vi "CountAtoms.vi"(0 "Cursor List":T2, 5 "Atom Image":dbl[][](graph), 7 "Experimental Variables":T1={"Pixel Size before binning (µm)"=6.0, "Imaging Wavelength (m)"=4.61e-07, "Isotope"=84, "1P1 Linewidth (MHz)"=30.5, "Imaging Detuning (MHz)"=0.0, "Software Bin Size"=1} {"Software Bin Size" items=["1"=1, "2"=2, "3"=3, "4"=4, "5"=5, "6"=6, "7"=7, "8"=8]; "Isotope" min=84 max=88; "Imaging Wavelength (m)" format="%#_6p"}, 9 "Background Image":dbl[][](graph), 11 "Drop Time":dbl=1e-06 min=1e-06 format="%#_6p") -> (4 "Number":dbl, 6 "OD":dbl[][](graph), 8 "Data Cuts":dbl[][](graph), 10 "Temperature (K) x":dbl format="%#_6p", 15 "Temperature (K) y":dbl format="%#_6p")   [LabVIEW 2015]
uses:
  <vilib>/Utility/miscctls.llb/LVCursorListTypeDef.ctl
  Controls/ExperimentParameters/experimentalvariables.ctl
  <vilib>/Utility/file.llb/Write Delimited Spreadsheet (DBL).vi
  <vilib>/Utility/file.llb/Read Delimited Spreadsheet (DBL).vi
panel:
  out "standard output":string
  out "standard error":string
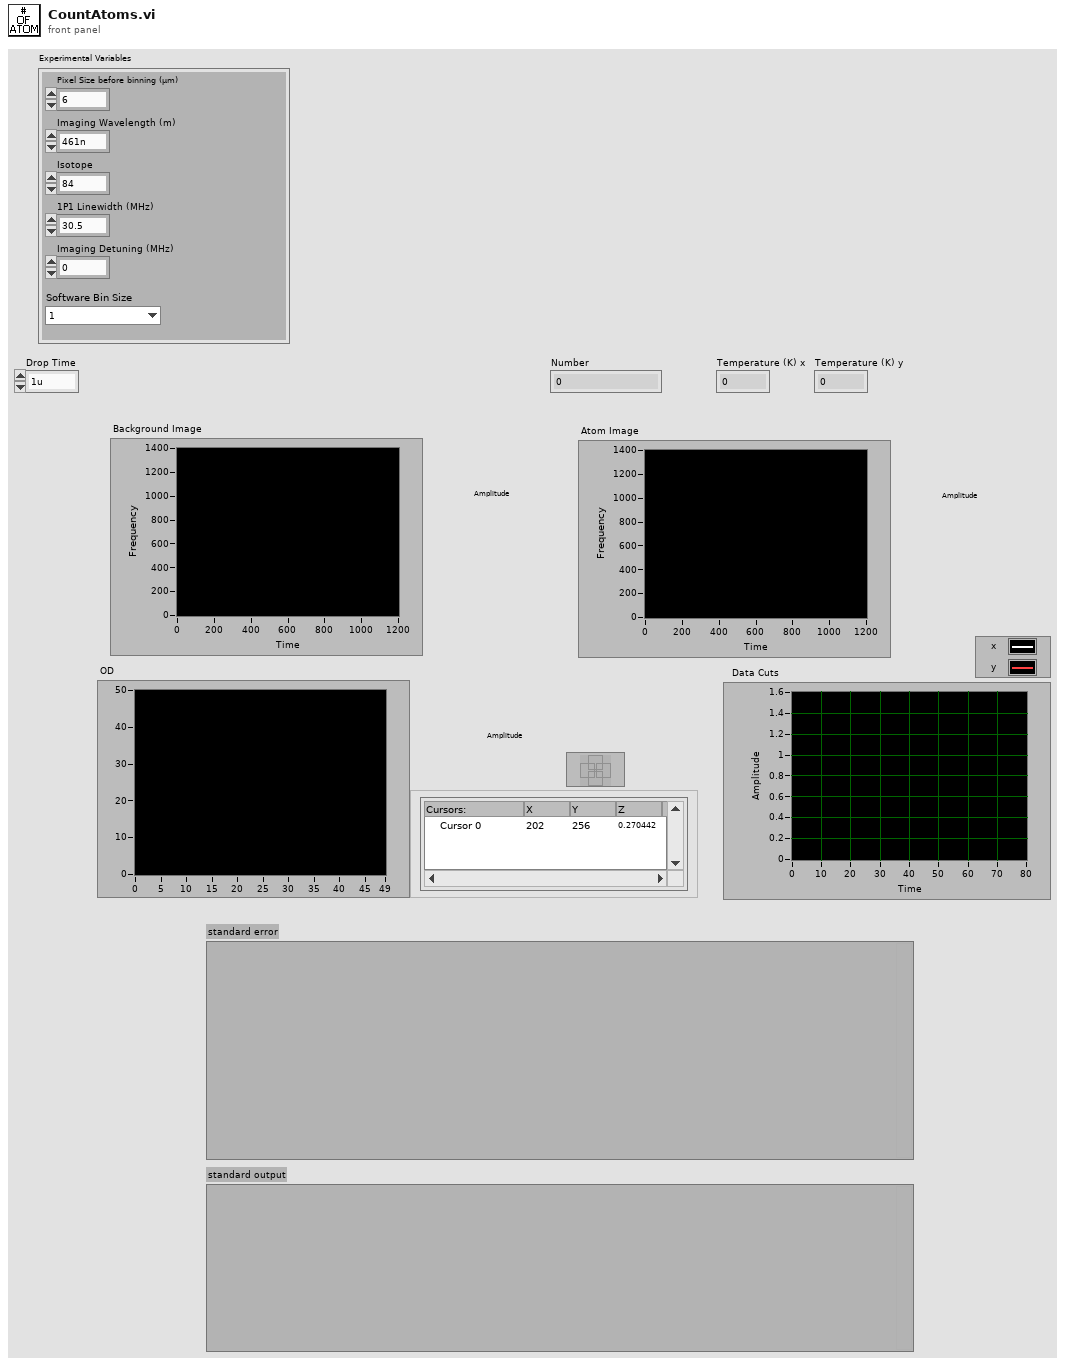
[diagram p1: front panel]
types:
  T1 = typedef "experimentalvariables.ctl" = cluster{"Pixel Size before binning (µm)":dbl, "Imaging Wavelength (m)":dbl, "Isotope":i32, "1P1 Linewidth (MHz)":dbl, "Imaging Detuning (MHz)":dbl, "Software Bin Size":u16}
  T2 = typedef "LVCursorListTypeDef.ctl" = cluster{"Name":string, "Color":u32, "Style":u8, "Point Style":u8, "Name Visible":bool, "Allow Drag":bool, "Cursor Mode":u32, "Plot":i32, "Index":i32, "Position":cluster{"X":dbl, "Y":dbl}, "X Scale":u32, "Y Scale":u32, "Watch Plots":i32[], "Watch All Plots":bool, "Plot Area":i32, "Label Offset":cluster{"X":dbl, "Y":dbl}}[]
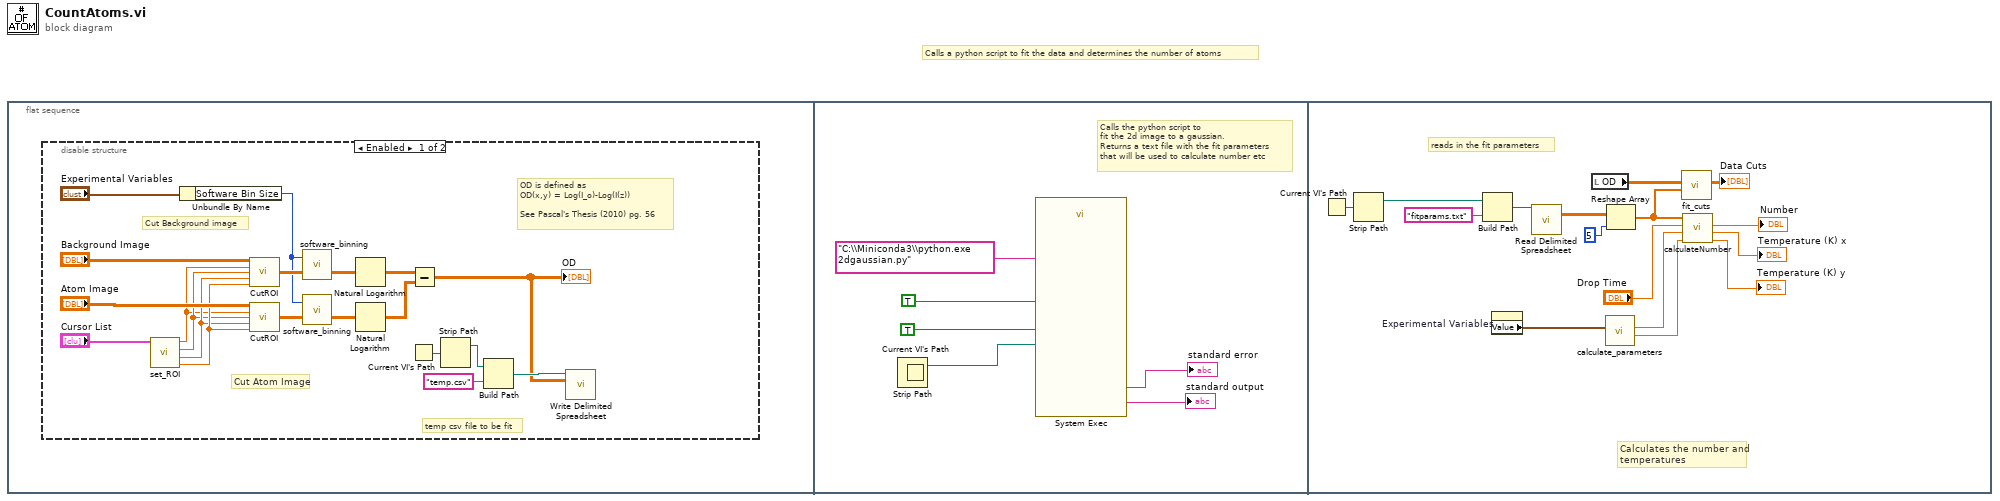
[diagram p0: block diagram]
diagram:
  # "Calls a python script to fit the data and determines the number of atoms"
  n1 = flat-sequence {
    frame #0 {
      n2 = disable-structure shown="Enabled" {
        frame Enabled {
          # "temp csv file to be fit"
          # "OD is defined as \nOD(x,y) = Log(I_o)-Log(I(z))\n\nSee Pascal's Thesis (2010) pg. 56"
          # "Cut Atom Image"
          # "Cut Background image"
          n3 = call "set_ROI.vi"("Cursor List"="Cursor List") -> ("Row End"=w15:dbl, "RowStart"=w14:dbl, "ColEnd"=w13:dbl, "ColStart"=w12:dbl)  [unwired: 7 in]
          n4 = Unbundle By Name("Experimental Variables") -> ("Software Bin Size"=w1:u16)
          n5 = call "CutROI.vi"("Full Image In"="Background Image", "Col Start"=w12, "Col End"=w13, "Row Start"=w14, "Row End"=w15) -> ("Cut Image Out"=w5:dbl[][])  [unwired: 10 in]
          n6 = call "CutROI.vi"("Full Image In"="Atom Image", "Col Start"=w12, "Col End"=w13, "Row Start"=w14, "Row End"=w15) -> ("Cut Image Out"=w3:dbl[][])  [unwired: 10 in]
          n7 = call "software_binning.vi"("Input Array"=w5, "bin size"=w1) -> ("Binned Array"=w4:dbl[][])  [unwired: 1 in]
          n8 = call "software_binning.vi"("Input Array"=w3, "bin size"=w1) -> ("Binned Array"=w2:dbl[][])  [unwired: 1 in]
          n9 = Natural Logarithm(1:w4) -> (0:w17:dbl[][])
          n10 = Natural Logarithm(1:w2) -> (0:w16:dbl[][])
          n11 = Current VI's Path() -> (path=w10:path)
          n12 = Subtract(x=w17, y=w16) -> (x-y=w6:dbl[][])
          "OD" <- w6
          n13 = Strip Path(path=w10) -> (stripped path=w9:path)  [unwired: 1 out]
          n14 = Build Path(base path=w9, name or relative path="temp.csv") -> (appended path=w8:path)
          n15 = call-poly <vilib>:"Write Delimited Spreadsheet.vi"("file path (dialog if empty)"=w8, "2D data"=w6) -> ()  [unwired: 12 in, 2 out]
        }
        frame Disabled {
        }
      }
    }
    frame #1 {
      # "Calls the python script to\nfit the 2d image to a gaussian.\nReturns a text file with the fit parameters\nthat will be used to calculate number etc"
      n16 = Current VI's Path() -> (path=w23:path)
      n17 = Strip Path(path=w23) -> (stripped path=w22:path)  [unwired: 1 out]
      n18 = call <vilib>:"System Exec.vi"("run minimized? (F)"=TRUE, "wait until completion? (T)"=TRUE, "working directory"=w22, "command line"="C:\\Miniconda3\\python.exe 2dgaussian.py") -> ("standard error"=→"standard error":string, "standard output"=→"standard output":string)  [unwired: 4 in, 2 out]
    }
    frame #2 {
      # "Calculates the number and \ntemperatures"
      # "reads in the fit parameters"
      n19 = Current VI's Path() -> (path=w34:path)
      n20 = Strip Path(path=w34) -> (stripped path=w33:path)  [unwired: 1 out]
      n21 = Build Path(base path=w33, name or relative path="fitparams.txt") -> (appended path=w35:path)
      n22 = property on="Experimental Variables" class="Clust (strict)"() -> ("Value"=w30:T1)  [unwired: 2 in, 2 out]
      n23 = call-poly <vilib>:"Read Delimited Spreadsheet.vi"("file path (dialog if empty)"=w35) -> ("all rows"=w43:dbl[][])  [unwired: 9 in, 5 out]
      n24 = local read "OD"() -> (w38:dbl[][])
      n25 = call "calculate_parameters.vi"("Experimental Variables"=w30) -> ("Effective Pixel Size (µm)"=w28:dbl, "Cross Section (m^2)"=w29:dbl)  [unwired: 8 in, 1 out]
      n26 = Reshape Array(w43, 5 ("dimension size")) -> (w31:dbl[])
      n27 = call "fit_cuts.vi"("Array"=w31, "Intensity Graph"=w38) -> ("Waveform Graph"=→"Data Cuts":dbl[][])  [unwired: 9 in]
      n28 = call "calculateNumber.vi"("Array"=w31, "Drop Time (s)"="Drop Time", "abs cross section (um^2)"=w29, "pixel size (um)"=w28) -> ("Number"=→"Number":dbl, "Temperature (K) x"=→"Temperature (K) x":dbl, "Temperature (K) y"=→"Temperature (K) y":dbl)  [unwired: 4 in]
    }
  }
